vi "vmd_preview_stop.vi"(10 "COM":bool, 11 "VISA name":refnum<visa-resource-name>) -> (3 "return":i32)   [LabVIEW 2016]
panel:
  in  "tVdCmdHeader":T1={"byCmdType"=15, "bySubCmd"=2, "byPara"=0, "byAddr_h"=0, "byAddr_l"=0, "byAddr_ll"=0, "byLen_h"=0, "byLen_l"=0}
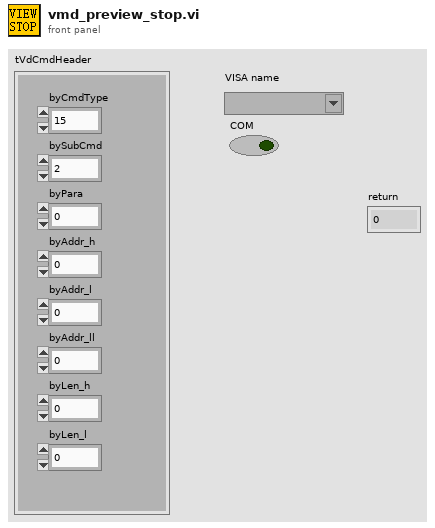
[diagram p1: front panel]
types:
  T1 = cluster{"byCmdType":u8, "bySubCmd":u8, "byPara":u8, "byAddr_h":u8, "byAddr_l":u8, "byAddr_ll":u8, "byLen_h":u8, "byLen_l":u8}
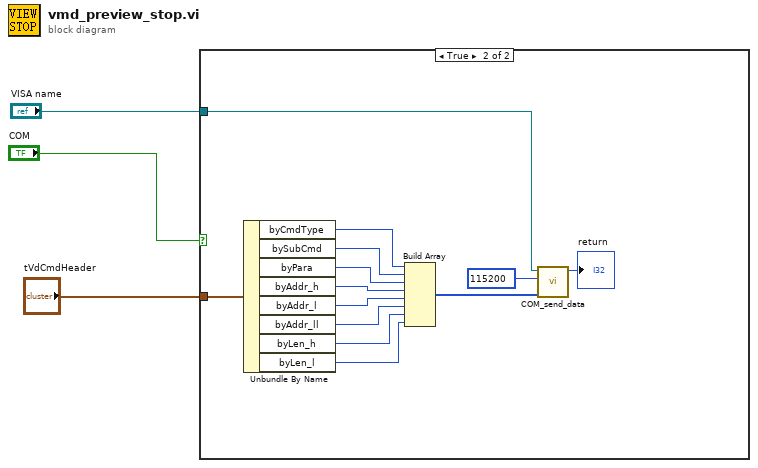
[diagram p0: block diagram]
diagram:
  n1 = case shown="True" "COM" {
    tunnel: "tVdCmdHeader" -> [_ w16]
    tunnel: "VISA name" -> [_ w7]
    frame False {
    }
    frame True {
      n2 = Unbundle By Name(w16) -> ("byCmdType"=w15:u8, "bySubCmd"=w14:u8, "byPara"=w13:u8, "byAddr_h"=w12:u8, "byAddr_l"=w11:u8, "byAddr_ll"=w10:u8, "byLen_h"=w9:u8, "byLen_l"=w8:u8)
      n3 = Build Array(w15, w14, w13, w12, w11, w10, w9, w8) -> (w6:u8[])
      n4 = call "COM_send_data.vi"("data"=w6, "baud rate (9600)"=u32 115200, "VISA name"=w7) -> ("return"=→"return":i32)  [unwired: 8 in]
    }
  }
